vi "Read Control Caption.vi"(8 "error in":errorcluster, 11 "Control Ref":refnum<vi>) -> (0 "error out":errorcluster, 2 "UTF-8 String":refnum<class "UTF-8 String.lvclass">)   [LabVIEW 2020, in "G-Unicode.lvlib"]
doc: "Reads text from a control or indicator, converting between encodings as necessary. <b>UTF-8 String</b> will be a scalar value, 1D array, or 2D array depending on <b>Control Ref</b> type.\n\nThe control text output will be converted to UTF-8 from either UTF-16LE or ANSI, depending on the control's Interpret As Unicode property or text Byte Order Mark (BOM).\n\nSupported control/indicator types and their outputs:\n- String (scalar)\n- String Array (1D)\n- String Array (2D)\n- Ring Text (1D)\n- Tab Pages (1D)\n- Boolean Text (1D, 4 elements)\n- Table (2D)\n- Listbox (1D)\n- Multicolumn Listbox (2D)"
uses:
  G-Unicode.lvlib
  18687cfd-7198-4a8c-9005-ae619691f07e.vi
  Types/UTF-8 String/UTF-8 String.lvclass
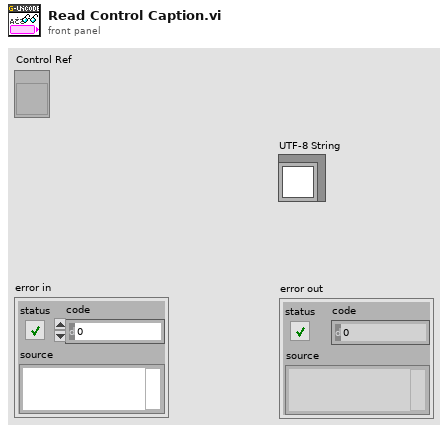
[diagram p1: front panel]
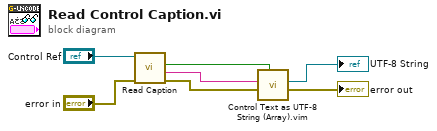
[diagram p0: block diagram]
diagram:
  n1 = call "Read Caption.vi"("error in"="error in", "Control Reference in"="Control Ref") -> ("error out"=w4:errorcluster, "Value"=w5:string, "Interpret As Unicode"=w2:bool)  [unwired: 6 in, 1 out]
  n2 = call "Control Text as UTF-8 String (Array).vim"("Interpret As Unicode"=w2, "error in"=w4, "Control Text"=w5) -> ("error out"=→"error out":errorcluster, "UTF-8 String"=→"UTF-8 String":refnum<class "UTF-8 String.lvclass">)  [unwired: 7 in]
